vi "test-swerve-drve-odometry-ALL.vi"(8 "error in (no error)":errorcluster) -> (0 "error out":errorcluster, 3 "ALL TEsts Passed":bool)   [LabVIEW 2019]
panel:
  out "Test 2":bool
  out "Test 1":bool
  out "Test 0":bool
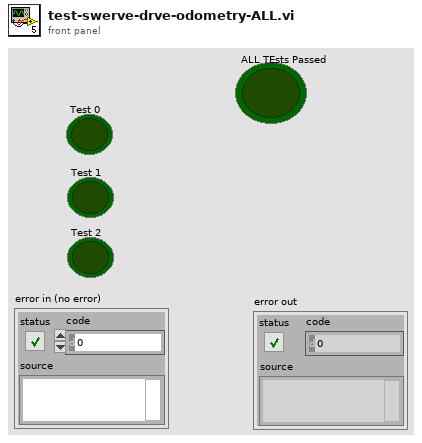
[diagram p1: front panel]
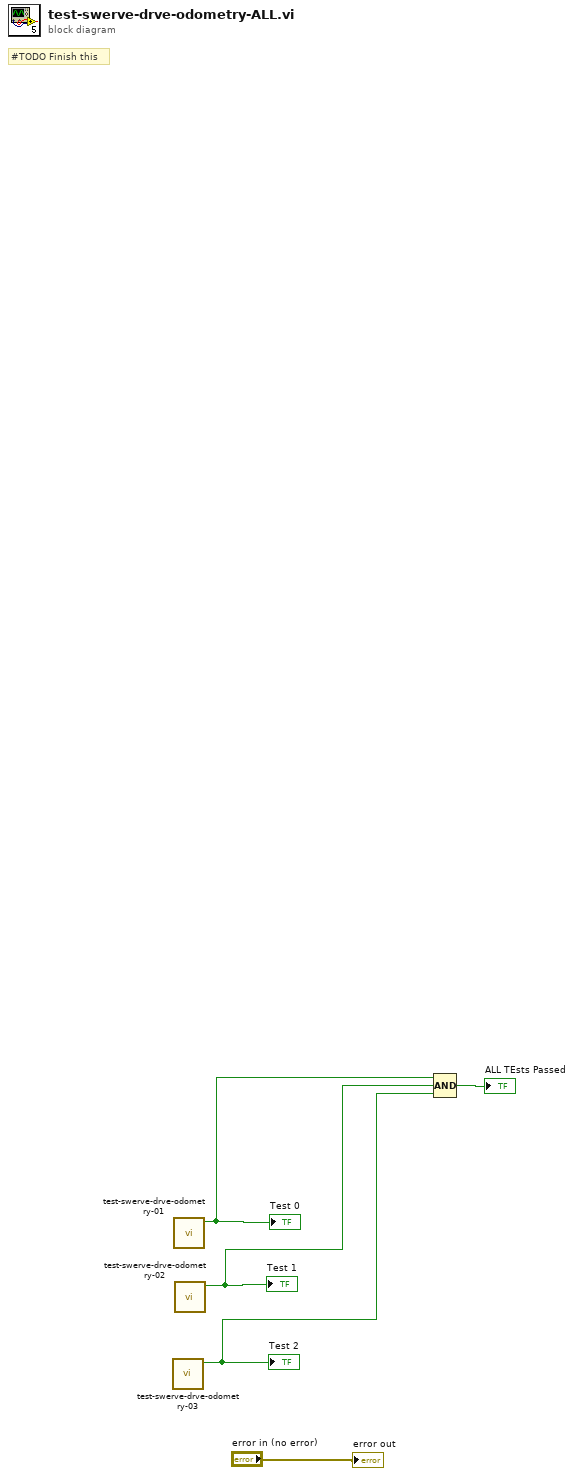
[diagram p0: block diagram]
diagram:
  # "#TODO Finish this"
  n1 = call "test-swerve-drve-odometry-03.vi"() -> ("Test Passed"=w3:bool)  [unwired: 11 in]
  "Test 2" <- w3
  n2 = call "test-swerve-drve-odometry-01.vi"() -> ("Test Passed"=w5:bool)  [unwired: 11 in]
  "Test 0" <- w5
  n3 = call "test-swerve-drve-odometry-02.vi"() -> ("Test Passed"=w4:bool)  [unwired: 11 in]
  "Test 1" <- w4
  n4 = Compound Arithmetic op=AND(w5, w4, w3) -> (→"ALL TEsts Passed":bool)
  "error out" <- "error in (no error)"
